vi "Fire_alarm_LABVIEW.vi"() -> ()   [LabVIEW 2020]
panel:
  in  "Table Control":string[][](table)
  out "Humidity":bool
  out "Temperature":bool
  out "Temp":dbl(slide) scale=0.0..50.0
  out "Humidity Chart":dbl(graph)
  out "Temperature Chart":dbl(graph)
  out "Humidity":dbl(knob) scale=0.0..100.0
  in  "VISA resource name":refnum<visa-resource-name>
  out "Gas Chart":dbl(graph)
  out "Gas":bool
  out "Fire Indicator":bool
  out "Gas":dbl(slide) scale=0.0..1.0
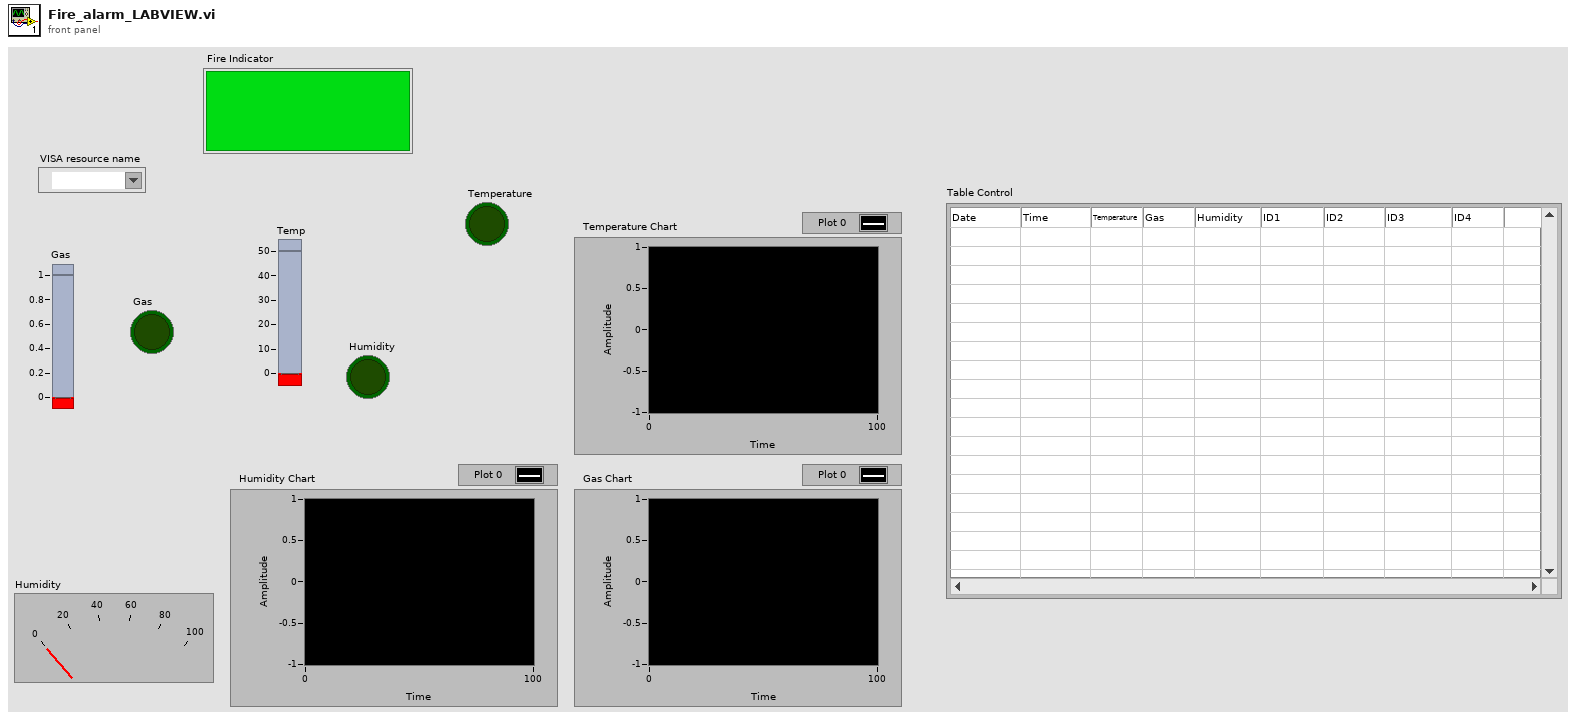
[diagram p1: front panel]
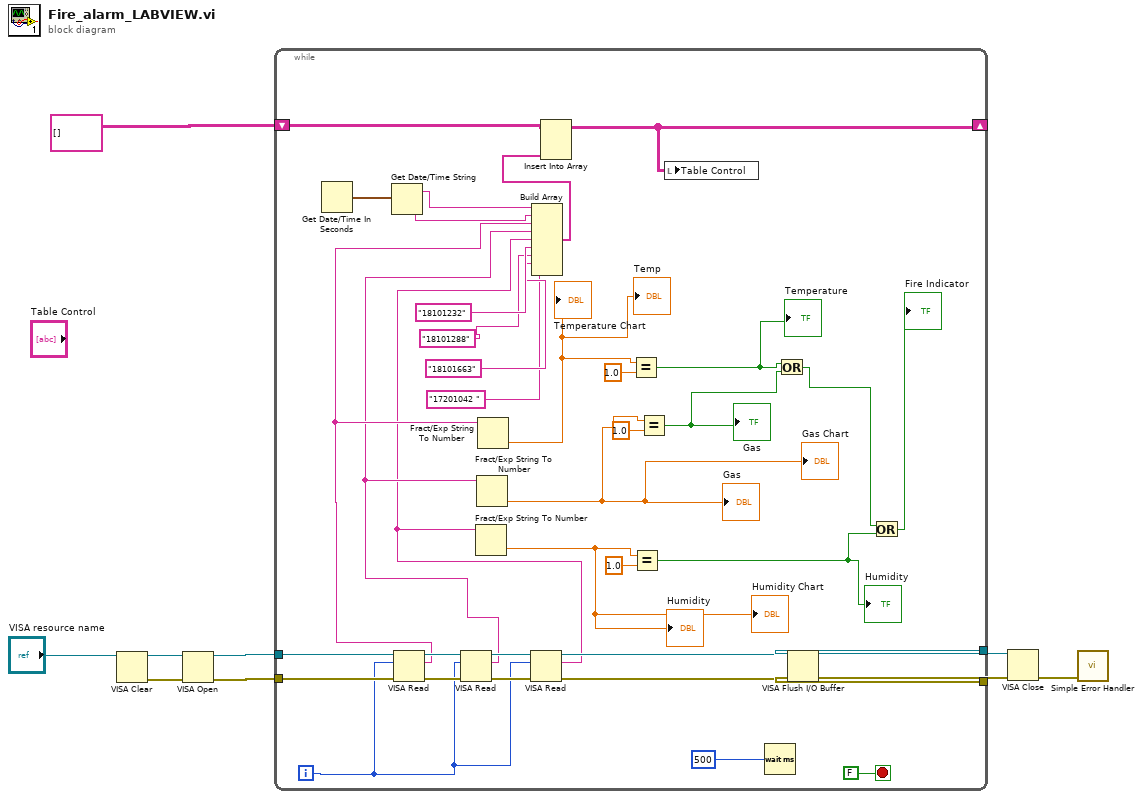
[diagram p0: block diagram]
diagram:
  n1 = VISA Clear(VISA resource name="VISA resource name") -> (VISA resource name out=w9:refnum<visa-resource-name>, error out=w8:errorcluster)  [unwired: 1 in]
  n2 = VISA Open(error in (no error)=w8, VISA resource name=w9) -> (VISA resource name=w7:refnum<visa-resource-name>, error out=w6:errorcluster)  [unwired: 3 in]
  n3 = while {
    tunnel: w7 -> [w46]
    tunnel: w6 -> [w45]
    tunnel: [w42] -> w5
    tunnel: [w41] -> w4
    shift-right: [w38] -> _
    shift-left: string[][] [] -> [w39]
    i -> [w22]
    stop <- FALSE stop-if-true
    n4 = Get Date/Time In Seconds() -> (seconds since 1Jan1904=w37:timestamp)
    n5 = Get Date/Time String(seconds (now)=w37) -> (date string=w36:string, time string=w35:string)  [unwired: 2 in]
    n6 = VISA Read(VISA resource name=w46, byte count=w22, error in (no error)=w45) -> (VISA resource name out=w44:refnum<visa-resource-name>, read buffer=w21:string, error out=w43:errorcluster)  [unwired: 1 out]
    n7 = VISA Read(VISA resource name=w44, byte count=w22, error in (no error)=w43) -> (VISA resource name out=w26:refnum<visa-resource-name>, read buffer=w20:string, error out=w25:errorcluster)  [unwired: 1 out]
    n8 = Fract/Exp String To Number(string=w20) -> (number=w30:dbl)  [unwired: 3 in, 1 out]
    "Gas Chart" <- w30
    "Gas" <- w30
    n9 = Fract/Exp String To Number(string=w21) -> (number=w27:dbl)  [unwired: 3 in, 1 out]
    "Temp" <- w27
    "Temperature Chart" <- w27
    n10 = VISA Read(VISA resource name=w26, byte count=w22, error in (no error)=w25) -> (VISA resource name out=w23:refnum<visa-resource-name>, read buffer=w19:string, error out=w24:errorcluster)  [unwired: 1 out]
    n11 = Fract/Exp String To Number(string=w19) -> (number=w17:dbl)  [unwired: 3 in, 1 out]
    "Humidity" <- w17
    "Humidity Chart" <- w17
    n12 = Build Array(w36, w35, w21, w20, w19, "18101232" ("element"), "18101288" ("element"), "18101663" ("element"), "17201042 " ("element")) -> (w34:string[])
    n13 = Insert Into Array(array=w39, new element=w34) -> (w38:string[][])  [unwired: 2 in]
    n14 = Equal?(x=w27, y=1.0) -> (x = y?=w28:bool)
    "Temperature" <- w28
    n15 = Equal?(x=w17, y=1.0) -> (x = y?=w16:bool)
    "Humidity" <- w16
    n16 = Equal?(x=w30, y=1.0) -> (x = y?=w29:bool)
    "Gas" <- w29
    n17 = local write "Table Control"(w38) -> ()
    n18 = Wait (ms)(milliseconds to wait=u32 500) -> ()  [unwired: 1 out]
    n19 = Or(x=w28, y=w29) -> (x .or. y?=w15:bool)
    n20 = VISA Flush I/O Buffer(VISA resource name=w23, error in (no error)=w24) -> (VISA resource name out=w42:refnum<visa-resource-name>, error out=w41:errorcluster)  [unwired: 1 in]
    n21 = Or(x=w15, y=w16) -> (x .or. y?=→"Fire Indicator":bool)
  }
  n22 = VISA Close(VISA resource name=w5, error in (no error)=w4) -> (error out=w3:errorcluster)
  n23 = call <vilib>:"Simple Error Handler.vi"("error in (no error)"=w3) -> ()  [unwired: 4 in, 5 out]
